vi "xmlFeature1.vi"(10 "Numeric":i32, 11 "Array":string[](array[string])) -> ()   [LabVIEW 2018]
uses:
  Global Variables.vi
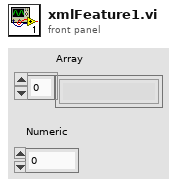
[diagram p1: front panel]
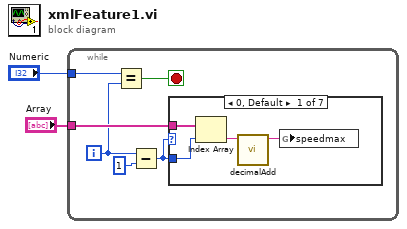
[diagram p0: block diagram]
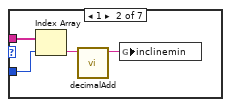
[diagram p2: hidden frame]
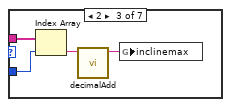
[diagram p3: hidden frame]
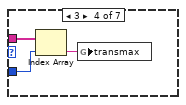
[diagram p4: hidden frame]
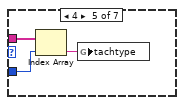
[diagram p5: hidden frame]
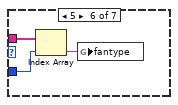
[diagram p6: hidden frame]
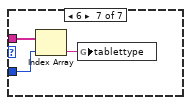
[diagram p7: hidden frame]
diagram:
  n1 = while {
    tunnel: "Array" -> [w8]
    tunnel: "Numeric" -> [w6]
    i -> [w4]
    stop <- w7 stop-if-true
    n2 = Equal?(x=w6, y=w4) -> (x = y?=w7:bool)
    n3 = Subtract(x=w4, y=1) -> (x-y=w5:i32)
    n4 = case shown="0, Default" w5 {
      tunnel: w8 -> [w12 w16 w19 w23 w26 w29 w32]
      tunnel: w5 -> [w10 w14 w18 w22 w25 w28 w31]
      frame 0, Default {
        n5 = Index Array(array=w12, index=w10) -> (element=w11:string)
        n6 = call "decimalAdd.vi"("inputString"=w11) -> ("resultString"=w9:string)  [unwired: 10 in]
        n7 = global write "Global Variables.vi" "speedmax"(w9) -> ()
      }
      frame 1 {
        n8 = Index Array(array=w16, index=w14) -> (element=w15:string)
        n9 = call "decimalAdd.vi"("inputString"=w15) -> ("resultString"=w13:string)  [unwired: 10 in]
        n10 = global write "Global Variables.vi" "inclinemin"(w13) -> ()
      }
      frame 2 {
        n11 = Index Array(array=w19, index=w18) -> (element=w20:string)
        n12 = call "decimalAdd.vi"("inputString"=w20) -> ("resultString"=w17:string)  [unwired: 10 in]
        n13 = global write "Global Variables.vi" "inclinemax"(w17) -> ()
      }
      frame 3 {
        n14 = Index Array(array=w23, index=w22) -> (element=w21:string)
        n15 = global write "Global Variables.vi" "transmax"(w21) -> ()
      }
      frame 4 {
        n16 = Index Array(array=w26, index=w25) -> (element=w24:string)
        n17 = global write "Global Variables.vi" "tachtype"(w24) -> ()
      }
      frame 5 {
        n18 = Index Array(array=w29, index=w28) -> (element=w27:string)
        n19 = global write "Global Variables.vi" "fantype"(w27) -> ()
      }
      frame 6 {
        n20 = Index Array(array=w32, index=w31) -> (element=w30:string)
        n21 = global write "Global Variables.vi" "tablettype"(w30) -> ()
      }
    }
  }
